vi "ZPL Config Continius.vi"(6 "Settle (1 mS)":u32=1, 8 "error":errorcluster, 10 "Continius (Default:0)":u16(ring) caption="INIT:CONTinius" items=["0", "1"], 11 "VISA":refnum<visa-resource-name>) -> (0 "error out":errorcluster={"status"=FALSE, "code"=-1073807346, "source"=""}, 3 "VISA out":refnum<visa-resource-name>)   [LabVIEW 2015]
doc: "If INIT:CONT is OFF, then INIT enables the trigger subsystem only for a single trigger action. The subsystem must be enabled prior to each subsequent trigger action. If INIT:CONT is ON, then the trigger system is continuously enabled and INIT is redundant.\n\nThis VI will wait for \"Settle\" milliseconds after setting the limit to allow the output to reach the new setting. If unwired, there will be no delay"
panel:
  # "Lambda ZPLUS \n Serial Port\n  DC Power Supplies"
  # "Transient Continius"
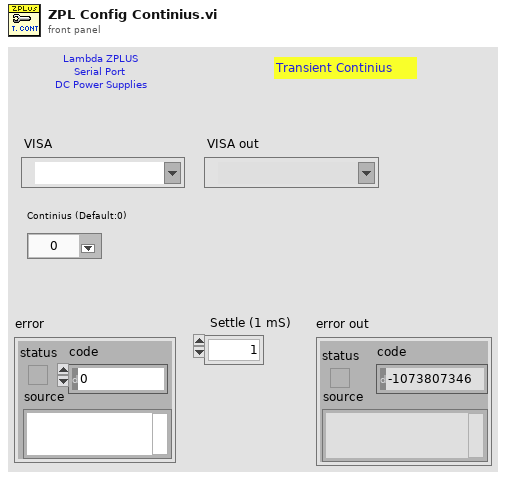
[diagram p1: front panel]
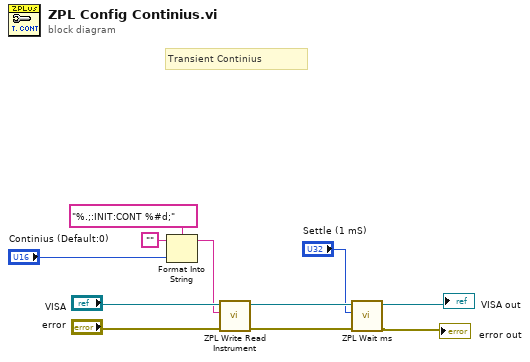
[diagram p0: block diagram]
diagram:
  # "Transient Continius"
  n1 = Format Into String(format string="%.;:INIT:CONT %#d;", initial string="", "Continius (Default:0)") -> (resulting string=w3:string)  [unwired: 1 in, 1 out]
  n2 = call "ZPL Write Read Instrument.vi"("error in"="error", "Write Command/Query SCPI"=w3, "VISA"="VISA") -> ("error out"=w8:errorcluster, "VISA  out"=w9:refnum<visa-resource-name>)  [unwired: 6 in, 1 out]
  n3 = call "ZPL Wait ms.vi"("error"=w8, "Delay (1 mS)"="Settle (1 mS)", "VISA"=w9) -> ("error out"=→"error out":errorcluster, "VISA out"=→"VISA out":refnum<visa-resource-name>)  [unwired: 7 in]
